vi "Apply Digital Out.vi"(8 "error in":errorcluster, 11 "DAQ970 in":refnum<class "DAQ970.lvclass">) -> (0 "error out":errorcluster, 3 "DAQ970 out":refnum<class "DAQ970.lvclass">)   [LabVIEW 2019, in "DAQ970.lvlib" / "DAQ970.lvclass"]
uses:
  Library/DAQ970.lvclass
  Library/DAQ970.lvclass/DAQ970.ctl
  <instrlib>/Keysight DAQ970/Keysight DAQ970.lvlib
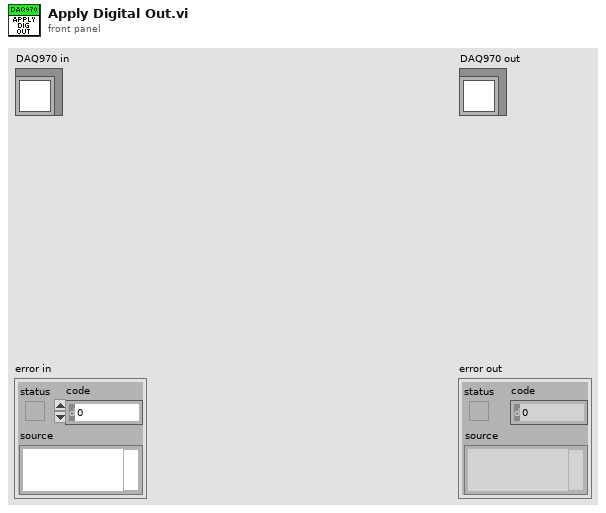
[diagram p1: front panel]
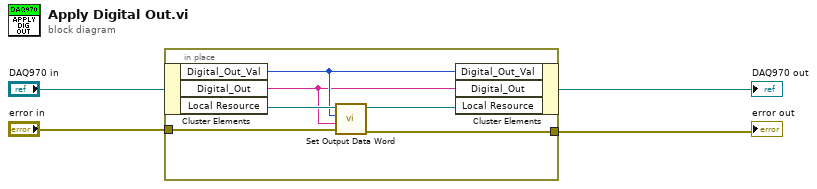
[diagram p0: block diagram]
diagram:
  n1 = in-place {
    in-place-border: "error in" -> [w8]
    in-place-border: [w7] -> w1
    n2 = in-place-cluster #1("DAQ970 in") -> ("Digital_Out_Val"=w6:u32, "Digital_Out"=w5:string, "Local Resource"=w10:refnum<k15>)
    n3 = call <instrlib>:"Set Output Data Word.vi"("error in (no error)"=w8, "ChannelList"=w5, "Data"=w6, "instrument handle"=w10) -> ("error out"=w7:errorcluster, "instrument handle out"=w9:refnum<k15>)  [unwired: 6 in]
    n4 = in-place-cluster #1("Digital_Out_Val"=w6, "Digital_Out"=w5, "Local Resource"=w9) -> (→"DAQ970 out":refnum<class "DAQ970.lvclass">)
  }
  "error out" <- w1
